vi "Convert to Units.vi"(8 "Fulcrum Ticks":dbl, 9 "Fulcrum Counts":dbl, 10 "Cart Ticks":dbl, 11 "Cart Counts":dbl) -> (0 "rad/sec":dbl, 1 "rad":dbl, 2 "meters/sec":dbl, 3 "meters":dbl)   [LabVIEW 2016]
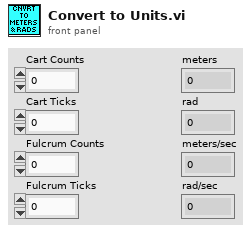
[diagram p1: front panel]
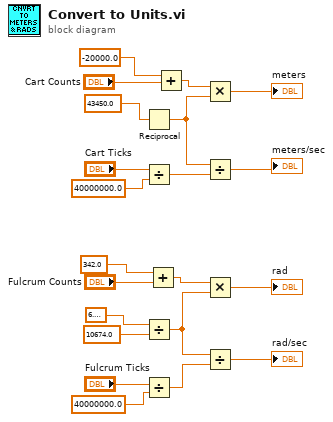
[diagram p0: block diagram]
diagram:
  n1 = Reciprocal(x=43450.0) -> (1/x=w7:dbl)
  n2 = Divide(x="Cart Ticks", y=40000000.0) -> (x/y=w10:dbl)
  n3 = Divide(x=6.283185307179586, y=10674.0) -> (x/y=w15:dbl)
  n4 = Divide(x="Fulcrum Ticks", y=40000000.0) -> (x/y=w16:dbl)
  n5 = Add(x=342.0, y="Fulcrum Counts") -> (x+y=w5:dbl)
  n6 = Add(x=-20000.0, y="Cart Counts") -> (x+y=w1:dbl)
  n7 = Multiply(x=w1, y=w7) -> (x*y=→"meters":dbl)
  n8 = Divide(x=w7, y=w10) -> (x/y=→"meters/sec":dbl)
  n9 = Multiply(x=w5, y=w15) -> (x*y=→"rad":dbl)
  n10 = Divide(x=w15, y=w16) -> (x/y=→"rad/sec":dbl)
